vi "Check Expression Errors.vi"(6 "For dialog?":bool, 7 "Expression String in":string, 8 "error in (no error)":errorcluster, 9 "Parser Error Details":T1, 10 "Found Variables":string[](array[string]), 11 "Expected Variables":string[](array[string])) -> (0 "error out":errorcluster)   [LabVIEW 2024, in "Output Sequencer.lvlib" / "Output Sequencer.lvclass"]
uses:
  Output Sequencer.lvclass
  Globals/Global Strings.vi
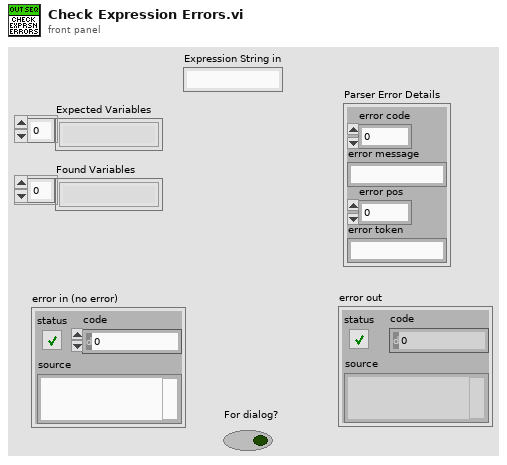
[diagram p1: front panel]
types:
  T1 = cluster{"error code":i32, "error message":string, "error pos":i32, "error token":string}
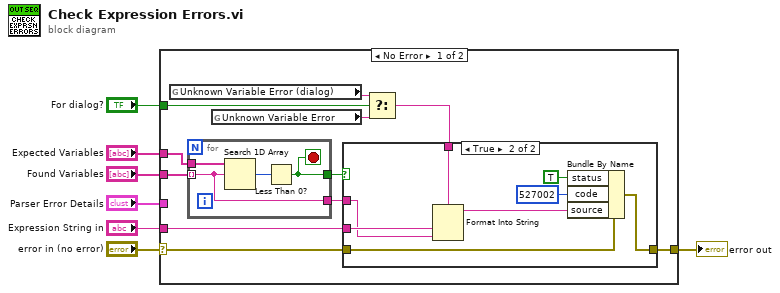
[diagram p0: block diagram]
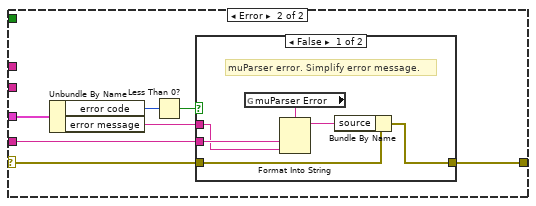
[diagram p3: hidden frame]
diagram:
  n1 = case shown="No Error" "error in (no error)" {
    selector: "error in (no error)" -> [w14 w35]
    tunnel: "Expression String in" -> [w18 w33]
    tunnel: "Found Variables" -> [w17 _]
    tunnel: "Expected Variables" -> [w16 _]
    tunnel: [w15 w34] -> w4
    tunnel: "Parser Error Details" -> [_ w38]
    tunnel: "For dialog?" -> [w9 _]
    frame No Error {
      n2 = global read "Global Strings.vi" "Unknown Variable Error (dialog)"() -> (w10:string)
      n3 = for {
        tunnel: w17 -> [w29] mode=indexing
        tunnel: w16 -> [w31]
        tunnel: [w29] -> w12
        tunnel: [w28] -> w13
        stop <- w28 stop-if-true
        n4 = Search 1D Array(1D array=w31, element=w29) -> (index of element=w30:i32)  [unwired: 1 in]
        n5 = Less Than 0?(x=w30) -> (x < 0?=w28:bool)
      }
      n6 = global read "Global Strings.vi" "Unknown Variable Error"() -> (w11:string)
      n7 = Select(t=w10, s=w9, f=w11) -> (s? t:f=w8:string)
      n8 = case shown="True" w13 {
        tunnel: w18 -> [_ w22]
        tunnel: [w19 w24] -> w15
        tunnel: w14 -> [w19 w23]
        tunnel: w12 -> [_ w21]
        tunnel: w8 -> [_ w20]
        frame False {
        }
        frame True {
          n9 = Format Into String(format string=w20, w22, w21) -> (resulting string=w27:string)  [unwired: 2 in, 1 out]
          n10 = Bundle By Name(cluster=w23, "status"=TRUE ("is warning? (False)"), "code"=527002 ("error code (0)"), "source"=w27) -> (w24:errorcluster)
        }
      }
    }
    frame Error {
      n11 = Unbundle By Name(w38) -> ("error code"=w37:i32, "error message"=w32:string)
      n12 = Less Than 0?(x=w37) -> (x < 0?=w36:bool)
      n13 = case shown="False" w36 {
        tunnel: w35 -> [w43 w45]
        tunnel: [w41 w45] -> w34
        tunnel: w33 -> [w40 _]
        tunnel: w32 -> [w39 _]
        frame False {
          # "muParser error. Simplify error message."
          n14 = global read "Global Strings.vi" "muParser Error"() -> (w44:string)
          n15 = Format Into String(format string=w44, w40, w39) -> (resulting string=w42:string)  [unwired: 2 in, 1 out]
          n16 = Bundle By Name(cluster=w43, "source"=w42) -> (w41:errorcluster)
        }
        frame True {
          # "Not a muParser LV API error. All error codes\nare positive (in range 515000-515102).\nPass existing error through."
        }
      }
    }
  }
  "error out" <- w4
